vi "ScanData.vi"(8 "ErrorIn":errorcluster, 11 "ScannedString":string) -> (0 "ErrorOut":errorcluster, 2 "Comment":string, 3 "Packets":T1[](array[typedef]))   [LabVIEW 2016]
doc: "Read important data coming from a text scanned from a file."
uses:
  FallSensor/Packet.ctl
  FallSensor/Sample.ctl
  FallSensor/Reading.ctl
  FallSensor/ReadingUnits/AccelReadingUnit.ctl
  FallSensor/ReadingUnits/GyroReadingUnit.ctl
  ScanDataContext.ctl
  FileSection.ctl
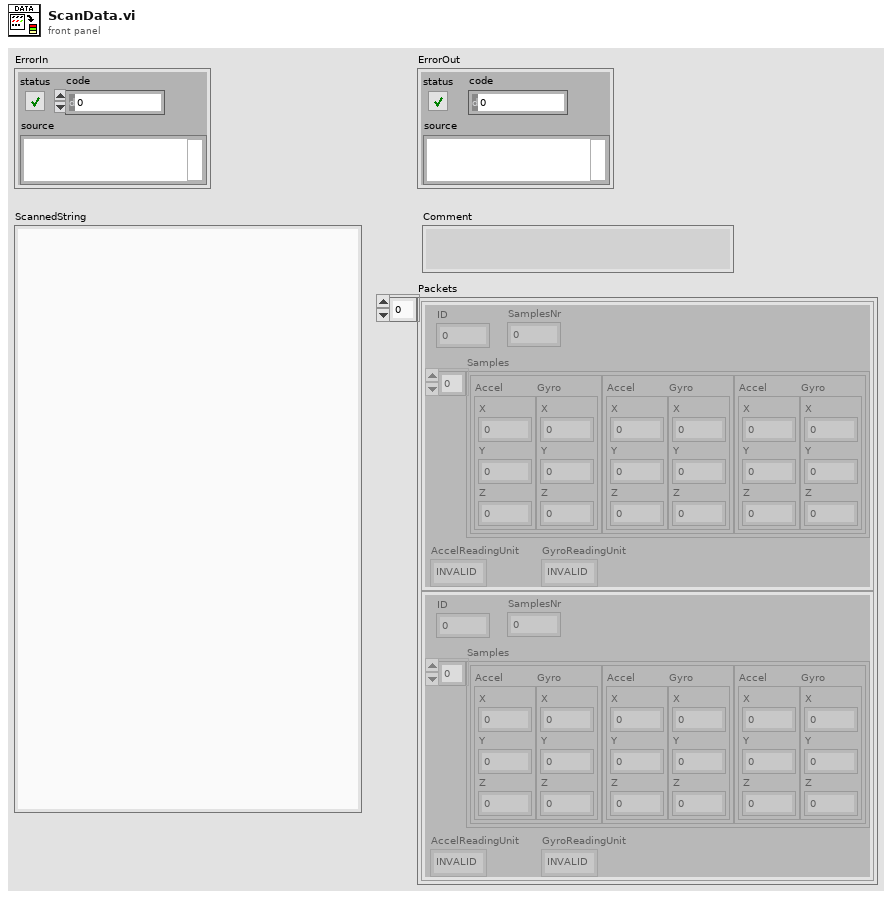
[diagram p1: front panel]
types:
  T1 = typedef "Packet.ctl" = cluster{"ID":u32, "SamplesNr":u32, "Samples":T2[], "AccelReadingUnit":T4, "GyroReadingUnit":T5}
  T2 = typedef "Sample.ctl" = cluster{"Accel":T3, "Gyro":T3}
  T3 = typedef "Reading.ctl" = cluster{"X":i16, "Y":i16, "Z":i16}
  T4 = typedef "AccelReadingUnit.ctl" = enum16{"INVALID", "RAW", "g"}
  T5 = typedef "GyroReadingUnit.ctl" = enum16{"INVALID", "RAW", "°/sec"}
  T6 = typedef "FileSection.ctl" = enum16{"SOF", "Header", "FileFormatVersion", "PacketsNumber", "Comment", "Data", "EOF"}
  T7 = typedef "ScanDataContext.ctl" = cluster{"HeaderSign":string, "LineOffset":i32, "SoughtPacketsNr":u16, "FileFormatVersion":string, "ScannedString":string, "Packets":T1[], "Comment":string}
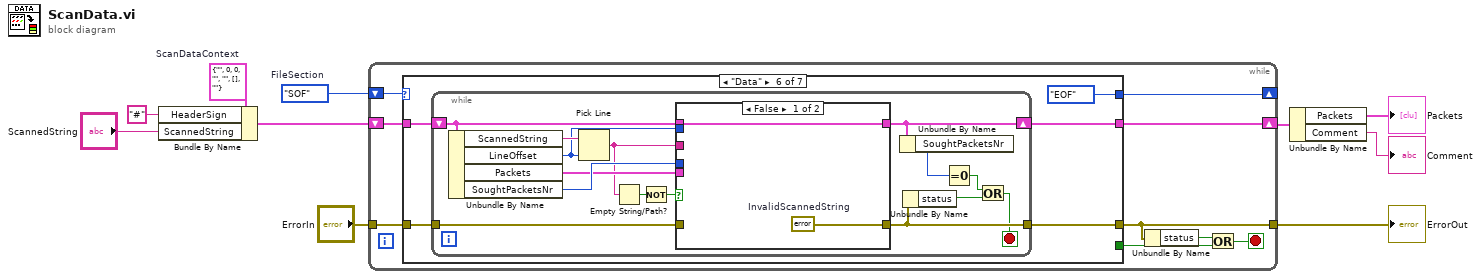
[diagram p0: block diagram]
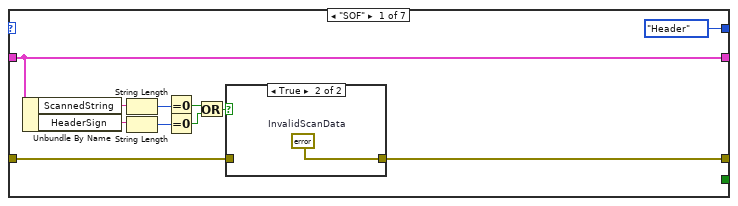
[diagram p2: hidden frame]
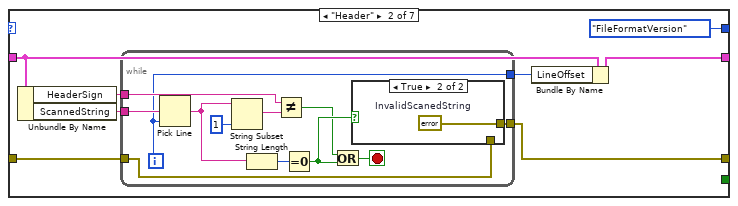
[diagram p4: hidden frame]
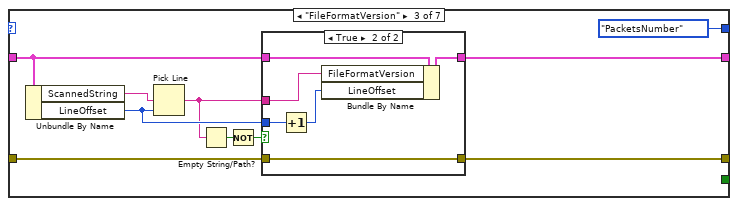
[diagram p6: hidden frame]
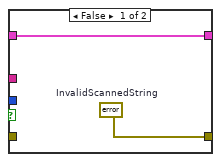
[diagram p7: hidden frame]
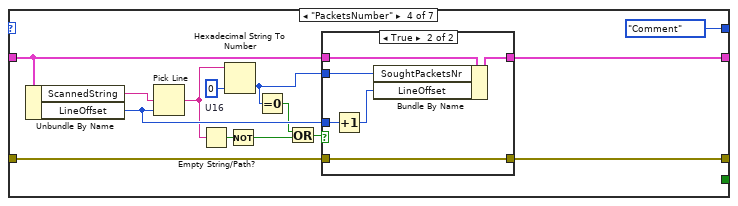
[diagram p8: hidden frame]
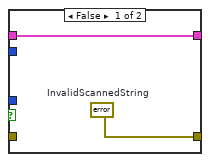
[diagram p9: hidden frame]
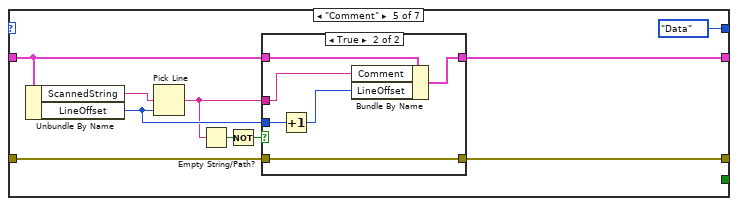
[diagram p10: hidden frame]
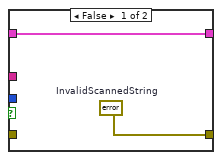
[diagram p11: hidden frame]
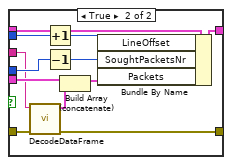
[diagram p12: hidden frame]
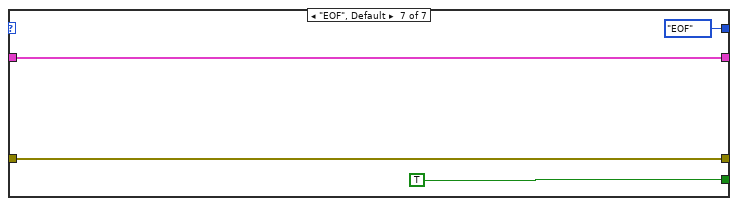
[diagram p13: hidden frame]
diagram:
  w8 = FileSection."SOF"  # FileSection
  w10 = T7 {"HeaderSign"="", "LineOffset"=0, "SoughtPacketsNr"=0, "FileFormatVersion"="", "ScannedString"="", "Packets"=[], "Comment"=""}  # ScanDataContext
  n1 = Bundle By Name(cluster=w10, "HeaderSign"="#", "ScannedString"="ScannedString") -> (w5:T7)
  n2 = while {
    shift-right: [w18] -> _
    shift-left: w8 -> [w19]
    tunnel: "ErrorIn" -> [w17]
    tunnel: [w13] -> w6
    shift-right: [w11] -> w4
    shift-left: w5 -> [w12]
    stop <- w14 stop-if-true
    n3 = case shown="\"Data\"" w19 {
      tunnel: [FileSection."Header" ("FileSection") FileSection."FileFormatVersion" ("FileSection") FileSection."PacketsNumber" ("FileSection") FileSection."Comment" ("FileSection") FileSection."Data" ("FileSection") FileSection."EOF" ("FileSection") FileSection."EOF" ("FileSection")] -> w18
      tunnel: [_ _ _ _ _ _ TRUE] -> w15
      tunnel: w17 -> [w27 w37 w61 w84 w101 w115 w148]
      tunnel: [w26 w38 w60 w83 w100 w114 w148] -> w13
      tunnel: w12 -> [w25 w35 w59 w82 w99 w117 w147]
      tunnel: [w25 w34 w58 w81 w98 w113 w147] -> w11
      frame "SOF" {
        n4 = Unbundle By Name(w25) -> ("ScannedString"=w23:string, "HeaderSign"=w29:string)
        n5 = String Length(string=w23) -> (length=w24:i32)
        n6 = String Length(string=w29) -> (length=w28:i32)
        n7 = Equal To 0?(x=w24) -> (x = 0?=w21:bool)
        n8 = Equal To 0?(x=w28) -> (x = 0?=w20:bool)
        n9 = Or(x=w21, y=w20) -> (x .or. y?=w22:bool)
        n10 = case shown="True" w22 {
          tunnel: w27 -> [w31 _]
          tunnel: [w31 w32] -> w26
          frame False {
          }
          frame True {
            w32 = errorcluster {"status"=TRUE, "code"=14, "source"="Invalid scan data"}  # InvalidScanData
          }
        }
      }
      frame "Header" {
        n11 = Unbundle By Name(w35) -> ("HeaderSign"=w36:string, "ScannedString"=w39:string)
        n12 = while {
          tunnel: w39 -> [w52]
          tunnel: [w50] -> w38
          tunnel: w37 -> [w49]
          tunnel: w36 -> [w45]
          tunnel: [w41] -> w33
          i -> [w41]
          stop <- w44 stop-if-true
          n13 = Pick Line(multi-line string=w52, line index=w41) -> (output string=w47:string)  [unwired: 1 in]
          n14 = String Subset(string=w47, length (rest)=1 ("length (rest)")) -> (substring=w46:string)  [unwired: 1 in]
          n15 = String Length(string=w47) -> (length=w51:i32)
          n16 = Not Equal?(x=w45, y=w46) -> (x != y?=w42:bool)
          n17 = Equal To 0?(x=w51) -> (x = 0?=w43:bool)
          n18 = Or(x=w42, y=w43) -> (x .or. y?=w44:bool)
          n19 = case shown="True" w43 {
            tunnel: [w53 w54] -> w50
            tunnel: w49 -> [w53 _]
            frame False {
            }
            frame True {
              w54 = errorcluster {"status"=TRUE, "code"=15, "source"="Invalid scanned string"}  # InvalidScanedString
            }
          }
        }
        n20 = Bundle By Name(cluster=w35, "LineOffset"=w33) -> (w34:T7)
      }
      frame "FileFormatVersion" {
        n21 = Unbundle By Name(w59) -> ("ScannedString"=w64:string, "LineOffset"=w56:i32)
        n22 = Pick Line(multi-line string=w64, line index=w56) -> (output string=w55:string)  [unwired: 1 in]
        n23 = Empty String/Path?(string/path=w55) -> (empty?=w63:bool)
        n24 = Not(x=w63) -> (.not. x?=w62:bool)
        n25 = case shown="True" w62 {
          tunnel: w61 -> [_ w72]
          tunnel: [w66 w72] -> w60
          tunnel: w55 -> [_ w69]
          tunnel: w59 -> [w65 w71]
          tunnel: [w65 w70] -> w58
          tunnel: w56 -> [_ w68]
          frame False {
            w66 = errorcluster {"status"=TRUE, "code"=14, "source"="Invalid scanned string"}  # InvalidScannedString
          }
          frame True {
            n26 = Increment(x=w68) -> (x+1=w67:i32)
            n27 = Bundle By Name(cluster=w71, "FileFormatVersion"=w69, "LineOffset"=w67) -> (w70:T7)
          }
        }
      }
      frame "PacketsNumber" {
        w78 = u16 0  # U16
        n28 = Unbundle By Name(w82) -> ("ScannedString"=w86:string, "LineOffset"=w79:i32)
        n29 = Pick Line(multi-line string=w86, line index=w79) -> (output string=w77:string)  [unwired: 1 in]
        n30 = Empty String/Path?(string/path=w77) -> (empty?=w85:bool)
        n31 = Hexadecimal String To Number(string=w77, default (0uL)=w78) -> (number=w73:u16)  [unwired: 1 in, 1 out]
        n32 = Not(x=w85) -> (.not. x?=w76:bool)
        n33 = Equal To 0?(x=w73) -> (x = 0?=w74:bool)
        n34 = Or(x=w74, y=w76) -> (x .or. y?=w75:bool)
        n35 = case shown="True" w75 {
          tunnel: w84 -> [_ w94]
          tunnel: [w88 w94] -> w83
          tunnel: w82 -> [w87 w93]
          tunnel: [w87 w92] -> w81
          tunnel: w79 -> [_ w91]
          tunnel: w73 -> [_ w89]
          frame False {
            w88 = errorcluster {"status"=TRUE, "code"=14, "source"="Invalid scanned string"}  # InvalidScannedString
          }
          frame True {
            n36 = Increment(x=w91) -> (x+1=w90:i32)
            n37 = Bundle By Name(cluster=w93, "SoughtPacketsNr"=w89, "LineOffset"=w90) -> (w92:T7)
          }
        }
      }
      frame "Comment" {
        n38 = Unbundle By Name(w99) -> ("ScannedString"=w104:string, "LineOffset"=w96:i32)
        n39 = Pick Line(multi-line string=w104, line index=w96) -> (output string=w95:string)  [unwired: 1 in]
        n40 = Empty String/Path?(string/path=w95) -> (empty?=w103:bool)
        n41 = Not(x=w103) -> (.not. x?=w102:bool)
        n42 = case shown="True" w102 {
          tunnel: w101 -> [_ w112]
          tunnel: [w106 w112] -> w100
          tunnel: w95 -> [_ w108]
          tunnel: w99 -> [w105 w111]
          tunnel: [w105 w110] -> w98
          tunnel: w96 -> [_ w109]
          frame False {
            w106 = errorcluster {"status"=TRUE, "code"=14, "source"="Invalid scanned string"}  # InvalidScannedString
          }
          frame True {
            n43 = Increment(x=w109) -> (x+1=w107:i32)
            n44 = Bundle By Name(cluster=w111, "Comment"=w108, "LineOffset"=w107) -> (w110:T7)
          }
        }
      }
      frame "Data" {
        n45 = while {
          shift-right: [w120] -> w113
          shift-left: w117 -> [w131]
          tunnel: w115 -> [w127]
          tunnel: [w125] -> w114
          stop <- w124 stop-if-true
          n46 = Unbundle By Name(w131) -> ("ScannedString"=w132:string, "LineOffset"=w130:i32, "Packets"=w122:T1[], "SoughtPacketsNr"=w123:u16)
          n47 = Pick Line(multi-line string=w132, line index=w130) -> (output string=w121:string)  [unwired: 1 in]
          n48 = Empty String/Path?(string/path=w121) -> (empty?=w129:bool)
          n49 = Not(x=w129) -> (.not. x?=w128:bool)
          n50 = case shown="False" w128 {
            tunnel: w131 -> [w133 w146]
            tunnel: [w133 w145] -> w120
            tunnel: w130 -> [_ w144]
            tunnel: w121 -> [_ w136]
            tunnel: w127 -> [_ w142]
            tunnel: [w134 w141] -> w125
            tunnel: w122 -> [_ w140]
            tunnel: w123 -> [_ w137]
            frame False {
              w134 = errorcluster {"status"=TRUE, "code"=14, "source"="Invalid scanned string"}  # InvalidScannedString
            }
            frame True {
              n51 = call "DecodeDataFrame.vi"("ErrorIn"=w142, "Frame"=w136) -> ("ErrorOut"=w141:errorcluster, "Packets"=w139:T1[])  [unwired: 8 in]
              n52 = Increment(x=w144) -> (x+1=w143:i32)
              n53 = Decrement(x=w137) -> (x-1=w135:u16)
              n54 = Build Array (concatenate)(w140, w139) -> (w138:T1[])
              n55 = Bundle By Name(cluster=w146, "LineOffset"=w143, "SoughtPacketsNr"=w135, "Packets"=w138) -> (w145:T7)
            }
          }
          n56 = Unbundle By Name(w120) -> ("SoughtPacketsNr"=w118:u16)
          n57 = Unbundle By Name(w125) -> ("status"=w126:bool)
          n58 = Equal To 0?(x=w118) -> (x = 0?=w119:bool)
          n59 = Or(x=w119, y=w126) -> (x .or. y?=w124:bool)
        }
      }
      frame "EOF", Default {
      }
    }
    n60 = Unbundle By Name(w13) -> ("status"=w16:bool)
    n61 = Or(x=w16, y=w15) -> (x .or. y?=w14:bool)
  }
  "ErrorOut" <- w6
  n62 = Unbundle By Name(w4) -> ("Packets"=→"Packets":T1[], "Comment"=→"Comment":string)
